vi "Serial Read Chart .vi"() -> ()   [LabVIEW 2016]
uses:
  <vilib>/Instr/_visa.llb/VISA Configure Serial Port (Instr).vi
panel:
  out "Waveform Chart":i32(graph)
  in  "VISA resource name":refnum<visa-resource-name>
  in  "stop":bool
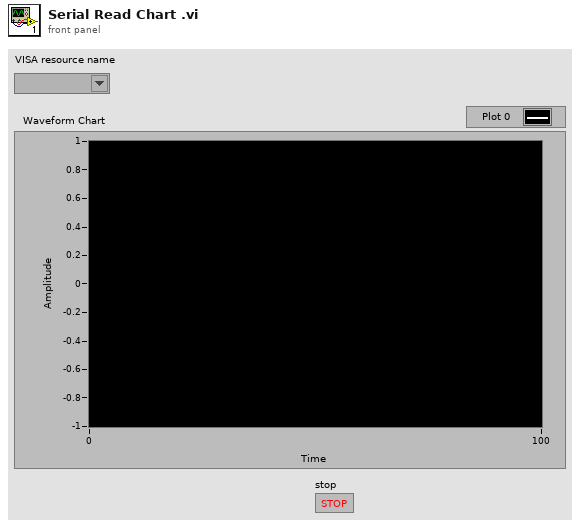
[diagram p1: front panel]
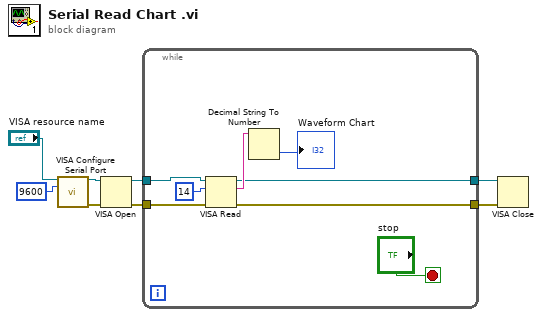
[diagram p0: block diagram]
diagram:
  n1 = call-poly "VISA Configure Serial Port"("VISA resource name"="VISA resource name", "baud rate (9600)"=u32 9600) -> ("VISA resource name out"=w7:refnum<visa-resource-name>, "error out"=w8:errorcluster)  [unwired: 12 in]
  n2 = VISA Open(error in (no error)=w8, VISA resource name=w7) -> (VISA resource name=w6:refnum<visa-resource-name>, error out=w5:errorcluster)  [unwired: 3 in]
  n3 = while {
    tunnel: w6 -> [w16]
    tunnel: w5 -> [w15]
    tunnel: [w11] -> w4
    tunnel: [w10] -> w3
    stop <- "stop" stop-if-true
    n4 = VISA Read(VISA resource name=w16, byte count=u32 14, error in (no error)=w15) -> (VISA resource name out=w10:refnum<visa-resource-name>, read buffer=w14:string, error out=w11:errorcluster)  [unwired: 1 out]
    n5 = Decimal String To Number(string=w14) -> (number=→"Waveform Chart":i32)  [unwired: 2 in, 1 out]
  }
  n6 = VISA Close(VISA resource name=w3, error in (no error)=w4) -> ()  [unwired: 1 out]
